vi "FPGA_convert_pannel-channel-to-U16-v1.vi"(1 "pannel|channel":u16) -> (0 "Numérique":u16)   [LabVIEW 2010]
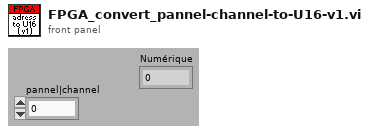
[diagram p1: front panel]
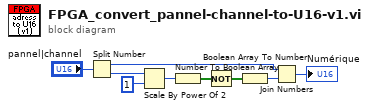
[diagram p0: block diagram]
diagram:
  n1 = Split Number(x="pannel|channel") -> (hi(x)=w4:u8, lo(x)=w1:u8)
  n2 = Scale By Power Of 2(n=w1, x=u8 1) -> (x*2^n=w6:u8)
  n3 = Number To Boolean Array(number=w6) -> (Boolean array=w7:bool[])
  n4 = Not(x=w7) -> (.not. x?=w8:bool[])
  n5 = Boolean Array To Number(Boolean array=w8) -> (number=w9:u8)
  n6 = Join Numbers(hi=w4, lo=w9) -> ((hi.lo)=→"Numérique":u16)
